vi "Myrio_TestMyrio.vi"() -> ()   [LabVIEW 2012]
uses:
  SubVIs/LVPresent_Globals.vi
panel:
  out "Z":dbl(slide) scale=0.0..16.0
  out "Y":dbl(slide) scale=0.0..16.0
  out "X":dbl(slide) scale=0.0..16.0
  in  "LED3":bool
  in  "LED1":bool
  in  "LED2":bool
  in  "LED0":bool
  # "myRIO\n\nTry clicking the buttons below to turn on the user LEDs on the myRIO"
  # "These are the outputs of the three accelerometers inside the myRIO."
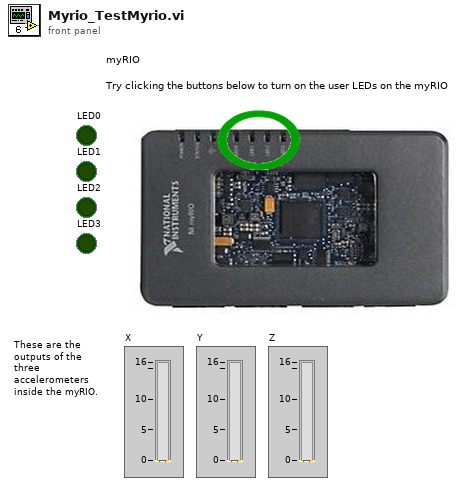
[diagram p1: front panel]
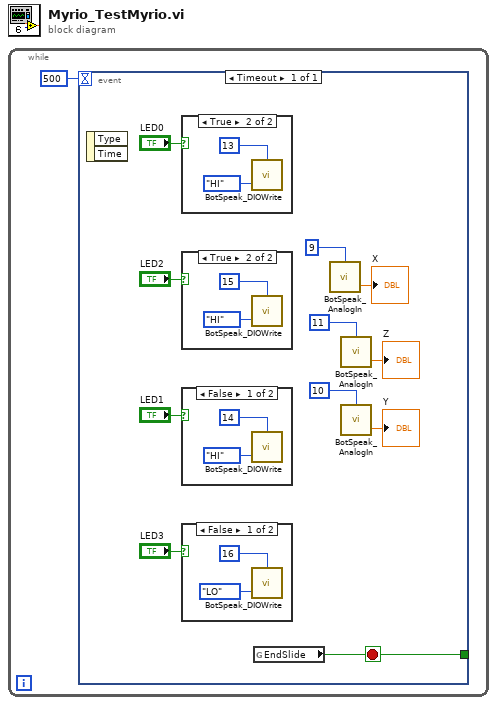
[diagram p0: block diagram]
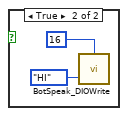
[diagram p2: hidden frame]
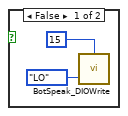
[diagram p3: hidden frame]
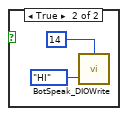
[diagram p4: hidden frame]
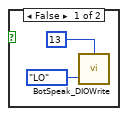
[diagram p5: hidden frame]
diagram:
  n1 = while {
    stop <- w2 stop-if-true
    n2 = event shown="[0] Timeout" {
      selector: _ -> [_]
      dyn-events: _ -> [_]
      timeout: 500 -> [_]
      tunnel: [w13] -> w2
      event Timeout {
        n3 = event-data() -> ()  [unwired: 1 in, 2 out]
        n4 = case shown="True" "LED0" {
          frame False {
            n5 = call <userlib>:"BotSpeak_DIOWrite.vi"("State"=enum32{"LO", "HI"}."LO", "DIO Line"=u32 13) -> ()  [unwired: 1 in, 2 out]
          }
          frame True {
            n6 = call <userlib>:"BotSpeak_DIOWrite.vi"("State"=enum32{"LO", "HI"}."HI", "DIO Line"=u32 13) -> ()  [unwired: 1 in, 2 out]
          }
        }
        n7 = case shown="True" "LED2" {
          frame False {
            n8 = call <userlib>:"BotSpeak_DIOWrite.vi"("State"=enum32{"LO", "HI"}."LO", "DIO Line"=u32 15) -> ()  [unwired: 1 in, 2 out]
          }
          frame True {
            n9 = call <userlib>:"BotSpeak_DIOWrite.vi"("State"=enum32{"LO", "HI"}."HI", "DIO Line"=u32 15) -> ()  [unwired: 1 in, 2 out]
          }
        }
        n10 = case shown="False" "LED1" {
          frame False {
            n11 = call <userlib>:"BotSpeak_DIOWrite.vi"("State"=enum32{"LO", "HI"}."HI", "DIO Line"=u32 14) -> ()  [unwired: 1 in, 2 out]
          }
          frame True {
            n12 = call <userlib>:"BotSpeak_DIOWrite.vi"("State"=enum32{"LO", "HI"}."HI", "DIO Line"=u32 14) -> ()  [unwired: 1 in, 2 out]
          }
        }
        n13 = case shown="False" "LED3" {
          frame False {
            n14 = call <userlib>:"BotSpeak_DIOWrite.vi"("State"=enum32{"LO", "HI"}."LO", "DIO Line"=u32 16) -> ()  [unwired: 1 in, 2 out]
          }
          frame True {
            n15 = call <userlib>:"BotSpeak_DIOWrite.vi"("State"=enum32{"LO", "HI"}."HI", "DIO Line"=u32 16) -> ()  [unwired: 1 in, 2 out]
          }
        }
        n16 = global read "LVPresent_Globals.vi" "EndSlide"() -> (w13:bool)
        n17 = call <userlib>:"BotSpeak_AnalogIn.vi"("A/D Channel"=u8 9) -> ("voltage"=→"X":dbl)  [unwired: 2 in, 1 out]
        n18 = call <userlib>:"BotSpeak_AnalogIn.vi"("A/D Channel"=u8 11) -> ("voltage"=→"Z":dbl)  [unwired: 2 in, 1 out]
        n19 = call <userlib>:"BotSpeak_AnalogIn.vi"("A/D Channel"=u8 10) -> ("voltage"=→"Y":dbl)  [unwired: 2 in, 1 out]
      }
    }
  }
